vi "SS2 Live_Filter Error.vi"(8 "error in (no error)":errorcluster, 11 "SS2 Q Elements in":T1[](array[typedef])) -> (0 "error out":errorcluster, 3 "SS2 Q Elements out":T1[](array[typedef]))   [LabVIEW 2019]
uses:
  SS2 Q [Element].ctl
  SS2 Q Event List.ctl
  SS2 Live_Settings List.ctl
  SS2 Live_Internal Data List.ctl
  Variant/Variant to Data/Variant to Data.lvlib
  Notebook/Notebook.lvlib
  Rich Text Box/Rich Text Box.lvlib
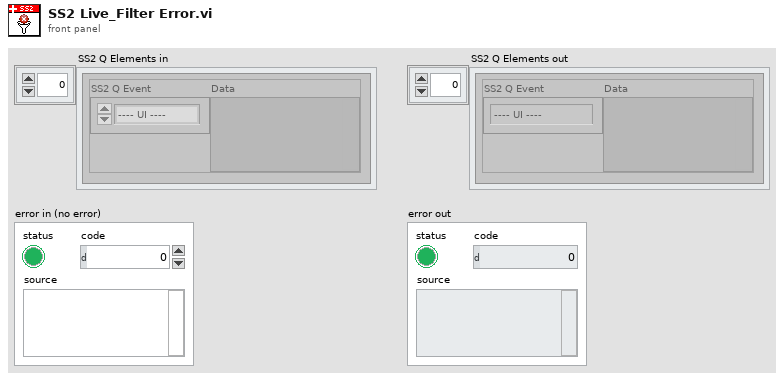
[diagram p1: front panel]
types:
  T1 = typedef "SS2 Q [Element].ctl" = cluster{"SS2 Q Event":T2, "Data":variant}
  T2 = typedef "SS2 Q Event List.ctl" = enum16{"---- UI ----", "Idle", "Initialization", "FPGA Status", "Reset FPGA", "Quit", "---- DAQ ----", "Start Recording", "Start Live Acquisition", "Initialize Recording Mode", "Initialize FPGA (Live Mode)", "Get Image Set", "Get Single Image", "Update Image Display", "Stop Live Acquisition", "Stop Data Recording", "Stop Data Saving", "---- Image ----", "Copy Data to Clipboard", "Set Image Palette", "Save Displayed Image with Overlay", "Save Image Data as TIFF"}
  T3 = typedef "SS2 Live_Settings List.ctl" = enum16{"FPGA:Bitfile Path", "FPGA:Bitfile Version", "FPGA:Auto Reset FPGA", "Acquisition Parameters:SS2 DAQ Parameters", "Acquisition Parameters:Gate Configuration Array", "Acquisition Parameters:Buffer Size (# Gates)", "File Information:File Information", "File Information:# Datasets in Series", "File Information:Scrambled File Flag", "File Information:Delay between Datasets", "Image Parameters:Image ROI Information", "Image Parameters:Image Binning Options", "UI Settings:Histogram Bins Number"}
  T4 = typedef "SS2 Live_Internal Data List.ctl" = enum16{"Number of pending file saving tasks", "File Saving Tasks Information", "Current Image ROI Information", "# FPGA Reset Attempts"}
  T5 = typedef "Rich Text Box.lvlib/Text Formatting.ctl" = cluster{"Font":string, "Text Color":T6, "Text Background Color":T6, "Text Style":enum16{"Regular", "Bold", "Italic", "Underline", "Strikeout"}, "Font Size (Points)":dbl, "Text Alignment":i32}
  T6 = typedef "Rich Text Box.lvlib/Text Colors.ctl" = enum16{"Unchanged", "Black", "Blue", "Gray", "Green", "Red", "White"}
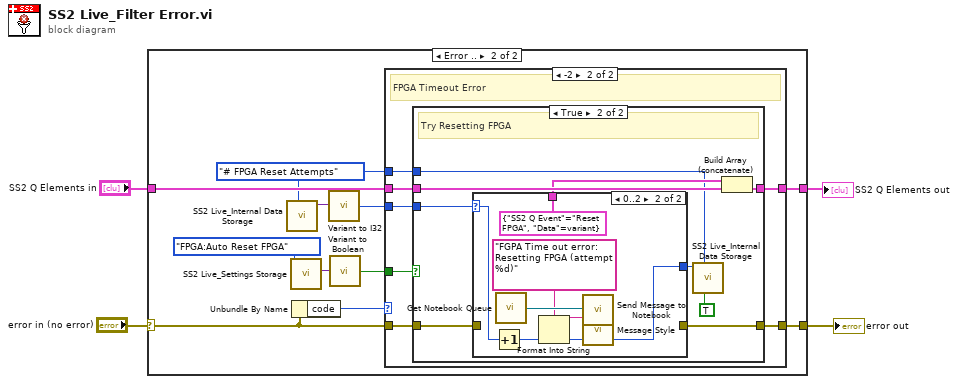
[diagram p0: block diagram]
diagram:
  n1 = case shown="Error .." "error in (no error)" {
    selector: "error in (no error)" -> [w5 w16]
    tunnel: "SS2 Q Elements in" -> [w6 w14]
    tunnel: [w6 w10] -> w2
    tunnel: [w5 w15] -> w1
    frame No Error {
    }
    frame Error {
      w7 = SS2_Live_Internal_Data_List."# FPGA Reset Attempts" ("SS2 Live Data")
      n2 = call "SS2 Live_Internal Data Storage.vi"("SS2 Live Data"=w7) -> ("Variant"=w9:variant)  [unwired: 8 in, 2 out]
      n3 = call "SS2 Live_Settings Storage.vi"("Settings List"=SS2_Live_Settings_List."FPGA:Auto Reset FPGA") -> ("Variant Data out"=w12:variant)  [unwired: 9 in, 1 out]
      n4 = Unbundle By Name(w16) -> ("code"=w17:i32)
      n5 = call "Variant to I32.vi"("Variant"=w9) -> ("Value"=w8:i32)  [unwired: 8 in]
      n6 = call "Variant to Boolean.vi"("Variant"=w12) -> ("Value"=w11:bool)  [unwired: 8 in]
      n7 = case shown="-2" w17 {
        tunnel: w16 -> [w19 w23]
        tunnel: [w19 w22] -> w15
        tunnel: w14 -> [w18 w25]
        tunnel: w11 -> [_ w26]
        tunnel: [w18 w24] -> w10
        tunnel: w8 -> [_ w21]
        tunnel: w7 -> [_ w20]
        frame 0, Default {
        }
        frame -2 {
          # "FPGA Timeout Error"
          n8 = case shown="True" w26 {
            tunnel: w25 -> [w28 w37]
            tunnel: [w28 w36] -> w24
            tunnel: w23 -> [w27 w34]
            tunnel: [w27 w33] -> w22
            tunnel: w21 -> [_ w32]
            tunnel: w20 -> [_ w30]
            frame False {
            }
            frame True {
              # "Try Resetting FPGA"
              n9 = case shown="0..2" w32 {
                selector: w32 -> [_ w40]
                tunnel: [_ T1 {"SS2 Q Event"=enum."Reset FPGA", "Data"=variant} ("element")] -> w35
                tunnel: w34 -> [w38 _]
                tunnel: [w38 _] -> w33
                tunnel: [_ w39] -> w29
                frame 3, Default {
                  # "Don't reset if 3 attempts have been made"
                }
                frame 0..2 {
                  n10 = Increment(x=w40) -> (x+1=w39:i32)
                  n11 = call "Get Notebook Queue.vi"() -> ("Notebook Queue"=w43:refnum<queue>)  [unwired: 9 in]
                  n12 = Format Into String(format string="FGPA Time out error: Resetting FPGA (attempt %d)" ("Message"), w39) -> (resulting string=w41:string)  [unwired: 2 in, 1 out]
                  n13 = call "Message Style.vi"() -> ("Message Formatting"=w44:T5)
                  n14 = call "Send Message to Notebook.vi"("Notebook Queue"=w43, "Message"=w41, "Text Formatting"=w44) -> ()  [unwired: 16 in, 1 out]
                }
              }
              n15 = call "SS2 Live_Internal Data Storage.vi"("Get(F)/Set"=TRUE, "SS2 Live Data"=w30, "Variant"=w29) -> ()  [unwired: 6 in, 3 out]
              n16 = Build Array (concatenate)(w35, w37) -> (w36:T1[])
            }
          }
        }
      }
    }
  }
  "error out" <- w1
  "SS2 Q Elements out" <- w2
